vi "filter.vi"(8 "debug":bool, 9 "conf.valid":bool, 10 "conf":u64, 11 "reset":bool) -> (1 "Ready.for.OrderBook.Command.Input":bool, 2 "Ready.for.Configuration.Input":bool)   [LabVIEW 2022 SP3]
uses:
  filter.states.ctl
  filter.data.ctl
  filter.debug.ctl
  filter.debug.slot.ctl
  filter.data.scratch.ctl
  common/orderbook.command.ctl
  common/orderbook.command.type.ctl
  filter.memory.command.ctl
  ticker.slot.ctl
  order.slot.ctl
  filter.getstate.ctl
  filter.getstate.slot.ctl
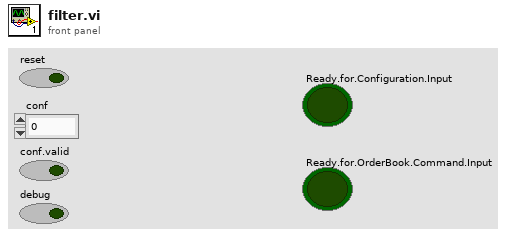
[diagram p1: front panel]
types:
  T1 = typedef "filter.data.ctl" = cluster{"filter.state":T2, "Debug":T3, "number.of.tickers":u32, "number.of.orders":u32, "filter.saved.state":T2, "Scratch":T5, "OrderBook.Command":T6, "Send.Command":bool, "memory.command":T8, "GetState":T11}
  T2 = typedef "filter.states.ctl" = enum16{"Noop", "Reset", "Debug", "Configuration", "Get.State", "Wait.for.Command", "Filter.Add", "Filter.Other", "Insert.Order", "Delete Order"}
  T3 = typedef "filter.debug.ctl" = cluster{"Write.to.Debug":bool, "debug.slot":T4}
  T4 = typedef "filter.debug.slot.ctl" = cluster{"Ticker":u64, "OrderId":u64}
  T5 = typedef "filter.data.scratch.ctl" = cluster{"I":u32, "N":u32, "Mode":u32, "OrderId":u64, "First Call?":bool, "Just Write":bool}
  T6 = typedef "orderbook.command.ctl" = cluster{"type":T7, "side":u8, "orderId ":u64, "quantity":u32, "symbol":u64, "price":u64, "executed.qty":u32, "canceled.qty":u32, "remaining.qty":u32, "seconds":u64, "nanoseconds":u64, "Add":bool, "Edit":bool, "Remove":bool}
  T7 = typedef "orderbook.command.type.ctl" = enum8{"Time", "AddOrder", "OrderExecuted", "OrderExecutedAtPrice", "ReduceSize", "ModifyOrder", "DeleteOrder", "Get.Everything", "Get.All.Orders", "Get.Top"}
  T8 = typedef "filter.memory.command.ctl" = cluster{"ticker.slot.value":T9, "order.slot.value":T10, "Write Ticker\nAddress":u32, "Write Ticker\nRequest":bool, "Read Ticker\nRequest":bool, "Read Ticker\nAddress":u32, "Read Ticker Valid":bool, "Write Order\nAddress":u32, "Write Order\nRequest":bool, "Read Order\nRequest":bool, "Read Order\nAddress":u32, "Read Order Valid":bool}
  T9 = typedef "ticker.slot.ctl" = cluster{"Symbol":u64}
  T10 = typedef "order.slot.ctl" = cluster{"OrderId":u64, "Quantity":u64}
  T11 = typedef "filter.getstate.ctl" = cluster{"Write.to.GetState":bool, "getstate.slot":T12}
  T12 = typedef "filter.getstate.slot.ctl" = cluster{"OrderId":u64, "Quantity":u64}
  T13 = cluster{"reset":bool, "conf":u64, "conf.valid":bool, "debug":bool}
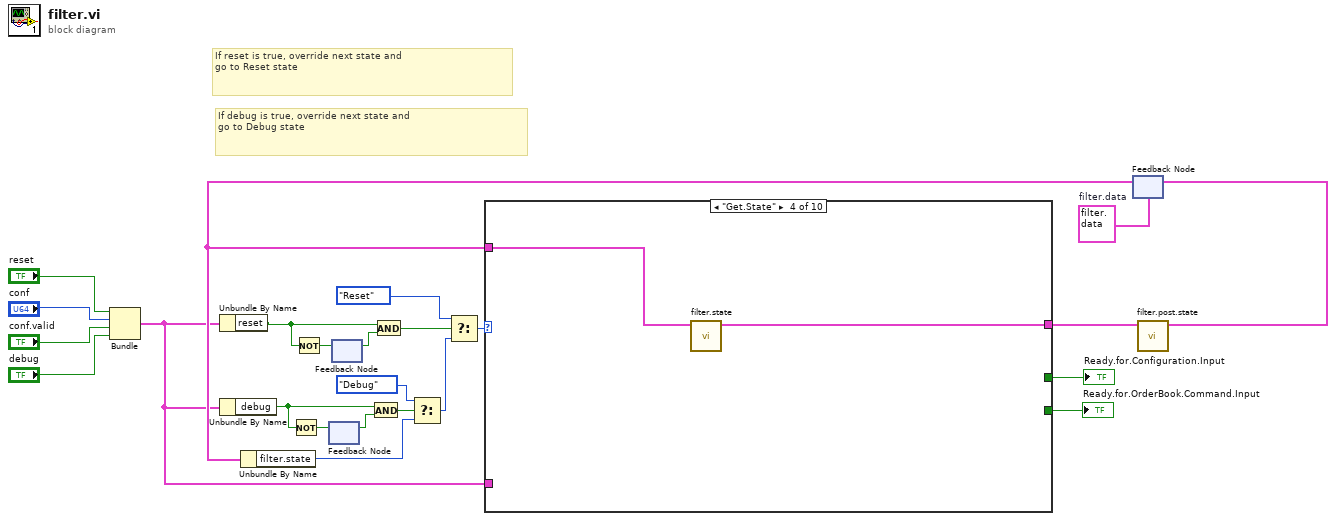
[diagram p0: block diagram]
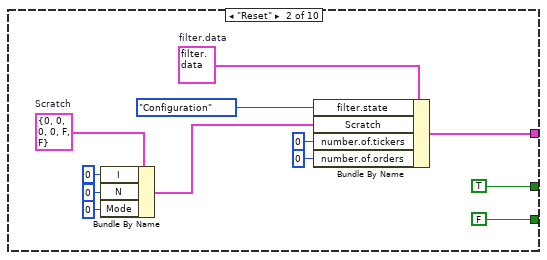
[diagram p3: hidden frame]
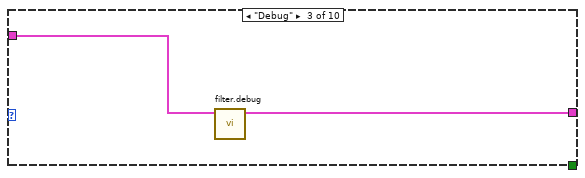
[diagram p4: hidden frame]
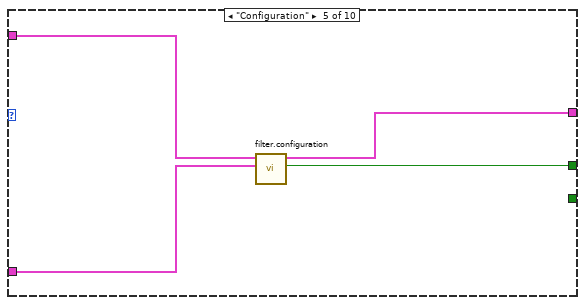
[diagram p5: hidden frame]
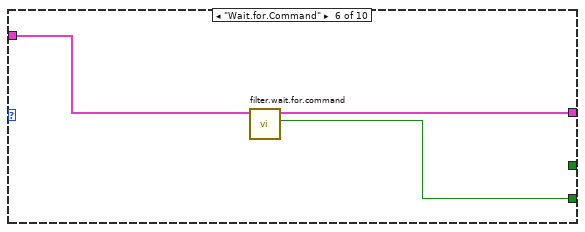
[diagram p6: hidden frame]
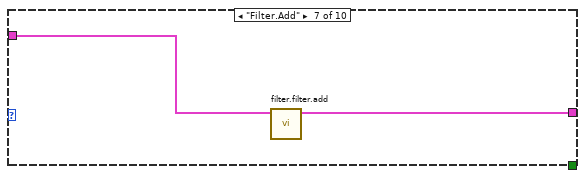
[diagram p7: hidden frame]
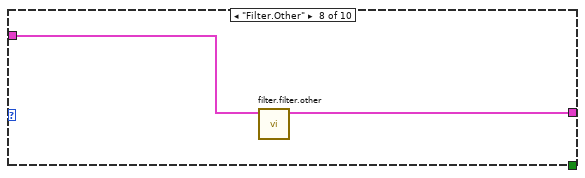
[diagram p8: hidden frame]
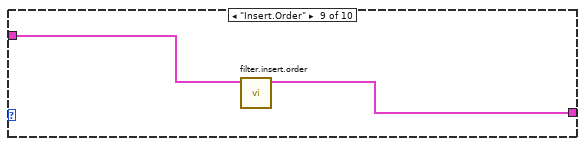
[diagram p9: hidden frame]
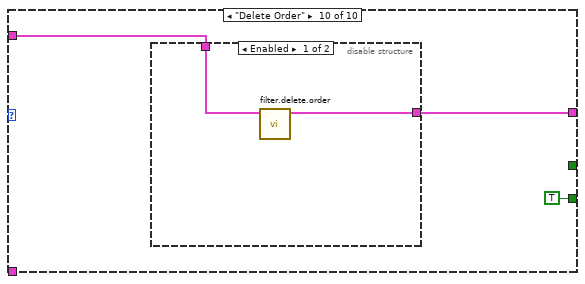
[diagram p10: hidden frame]
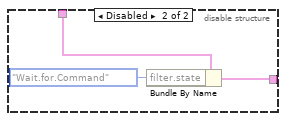
[diagram p11: hidden frame]
diagram:
  w9 = T1 {"filter.state"=enum."Noop", "Debug"={"Write.to.Debug"=FALSE, "debug.slot"={"Ticker"=0, "OrderId"=0}}, "number.of.tickers"=0, "number.of.orders"=0, "filter.saved.state"=enum."Noop", "Scratch"={"I"=0, "N"=0, "Mode"=0, "OrderId"=0, "First Call?"=FALSE, "Just Write"=FALSE}, "OrderBook.Command"={"type"=enum."Time", "side"=0, "orderId "=0, "quantity"=0, "symbol"=0, "price"=0, "executed.qty"=0, "canceled.qty"=0, "remaining.qty"=0, "seconds"=0, "nanoseconds"=0, "Add"=FALSE, "Edit"=FALSE, "Remove"=FALSE}, "Send.Command"=FALSE, "memory.command"={"ticker.slot.value"={"Symbol"=0}, "order.slot.value"={"OrderId"=0, "Quantity"=0}, "Write Ticker\nAddress"=0, "Write Ticker\nRequest"=FALSE, "Read Ticker\nRequest"=FALSE, "Read Ticker\nAddress"=0, "Read Ticker Valid"=FALSE, "Write Order\nAddress"=0, "Write Order\nRequest"=FALSE, "Read Order\nRequest"=FALSE, "Read Order\nAddress"=0, "Read Order Valid"=FALSE}, "GetState"={"Write.to.GetState"=FALSE, "getstate.slot"={"OrderId"=0, "Quantity"=0}}}  # filter.data
  # "If debug is true, override next state and \ngo to Debug state"
  # "If reset is true, override next state and \ngo to Reset state"
  n1 = Bundle("reset"="reset", "conf"="conf", "conf.valid"="conf.valid", "debug"="debug") -> (w3:T13)  [unwired: 1 in]
  n2 = Unbundle By Name(w3) -> ("reset"=w18:bool)
  n3 = Unbundle By Name(w3) -> ("debug"=w15:bool)
  n4 = Not(x=w15) -> (.not. x?=w17:bool)
  n5 = Not(x=w18) -> (.not. x?=w20:bool)
  n6 = feedback #1() -> (w16:bool)  [unwired: 1 in]
  n7 = feedback-in #1(w17) -> ()
  n8 = feedback #2() -> (w19:bool)  [unwired: 1 in]
  n9 = feedback-in #2(w20) -> ()
  n10 = And(x=w15, y=w16) -> (x .and. y?=w12:bool)
  n11 = And(x=w18, y=w19) -> (x .and. y?=w13:bool)
  n12 = feedback #3(w9) -> (w6:T1)
  n13 = Unbundle By Name(w6) -> ("filter.state"=w8:T2)
  n14 = Select(t=filter.states."Debug" ("filter.states"), s=w12, f=w8) -> (s? t:f=w10:T2)
  n15 = Select(t=filter.states."Reset" ("filter.states"), s=w13, f=w10) -> (s? t:f=w7:T2)
  n16 = case shown="\"Get.State\"" w7 {
    tunnel: [w25 w36 w39 w41 w45 w46 w50 w51 w53 w55] -> w1
    tunnel: w6 -> [w25 _ w38 w40 w43 w48 w49 w52 w54 w56]
    tunnel: [_ TRUE _ _ w42 _ _ _ _ _] -> w5
    tunnel: [_ FALSE _ _ _ w47 _ _ _ TRUE ("Ready.for.OrderBook.Command.Input")] -> w4
    tunnel: w3 -> [_ _ _ _ w44 _ _ _ _ _]
    frame "Noop", Default {
    }
    frame "Reset" {
      w32 = T5 {"I"=0, "N"=0, "Mode"=0, "OrderId"=0, "First Call?"=FALSE, "Just Write"=FALSE}  # Scratch
      w37 = T1 {"filter.state"=enum."Noop", "Debug"={"Write.to.Debug"=FALSE, "debug.slot"={"Ticker"=0, "OrderId"=0}}, "number.of.tickers"=0, "number.of.orders"=0, "filter.saved.state"=enum."Noop", "Scratch"={"I"=0, "N"=0, "Mode"=0, "OrderId"=0, "First Call?"=FALSE, "Just Write"=FALSE}, "OrderBook.Command"={"type"=enum."Time", "side"=0, "orderId "=0, "quantity"=0, "symbol"=0, "price"=0, "executed.qty"=0, "canceled.qty"=0, "remaining.qty"=0, "seconds"=0, "nanoseconds"=0, "Add"=FALSE, "Edit"=FALSE, "Remove"=FALSE}, "Send.Command"=FALSE, "memory.command"={"ticker.slot.value"={"Symbol"=0}, "order.slot.value"={"OrderId"=0, "Quantity"=0}, "Write Ticker\nAddress"=0, "Write Ticker\nRequest"=FALSE, "Read Ticker\nRequest"=FALSE, "Read Ticker\nAddress"=0, "Read Ticker Valid"=FALSE, "Write Order\nAddress"=0, "Write Order\nRequest"=FALSE, "Read Order\nRequest"=FALSE, "Read Order\nAddress"=0, "Read Order Valid"=FALSE}, "GetState"={"Write.to.GetState"=FALSE, "getstate.slot"={"OrderId"=0, "Quantity"=0}}}  # filter.data
      n17 = Bundle By Name(cluster=w32, "I"=u32 0, "N"=u32 0, "Mode"=u32 0) -> (w31:T5)
      n18 = Bundle By Name(cluster=w37, "filter.state"=filter.states."Configuration", "Scratch"=w31, "number.of.tickers"=u32 0, "number.of.orders"=u32 0) -> (w36:T1)
    }
    frame "Debug" {
      n19 = call "filter.debug.vi"("filter.data in"=w38) -> ("filter.data out"=w39:T1)  [unwired: 10 in]
    }
    frame "Get.State" {
      n20 = call "filter.state.vi"("filter.data in"=w40) -> ("filter.data out"=w41:T1)  [unwired: 10 in]
    }
    frame "Configuration" {
      n21 = call "filter.configuration.vi"("Cluster"=w44, "filter.data in"=w43) -> ("Boolean"=w42:bool, "filter.data out"=w45:T1)  [unwired: 8 in]
    }
    frame "Wait.for.Command" {
      n22 = call "filter.wait.for.command.vi"("filter.data in"=w48) -> ("Ready.for.OrderBook.Command.Input"=w47:bool, "filter.data out"=w46:T1)  [unwired: 9 in]
    }
    frame "Filter.Add" {
      n23 = call "filter.filter.add.vi"("filter.data in"=w49) -> ("filter.data out"=w50:T1)  [unwired: 10 in]
    }
    frame "Filter.Other" {
      n24 = call "filter.filter.other.vi"("filter.data in"=w52) -> ("filter.data out"=w51:T1)  [unwired: 10 in]
    }
    frame "Insert.Order" {
      n25 = call "filter.insert.order.vi"("filter.data in"=w54) -> ("filter.data out"=w53:T1)  [unwired: 10 in]
    }
    frame "Delete Order" {
      n26 = disable-structure shown="Enabled" {
        disable-tunnel: w56 -> [w59 w62]
        disable-tunnel: [w58 w61] -> w55
        frame Enabled {
          n27 = call "filter.delete.order.vi"("filter.data in"=w59) -> ("filter.data out"=w58:T1)  [unwired: 10 in]
        }
        frame Disabled {
          n28 = Bundle By Name(cluster=w62, "filter.state"=filter.states."Wait.for.Command") -> (w61:T1)
        }
      }
    }
  }
  "Ready.for.OrderBook.Command.Input" <- w4
  "Ready.for.Configuration.Input" <- w5
  n29 = call "filter.post.state.vi"("filter.data in"=w1) -> ("filter.data out 2"=w2:T1)  [unwired: 10 in]
  n30 = feedback-in #3(w2) -> ()
